vi "AddChannel.vi"(0 "VIRef":refnum<vi>[](array[refnum]), 1 "Name":string="172.16.21.19", 3 "SetCurrent":dbl format="%#.2g", 5 "ADRESS":string[](array[string]), 7 "error in (no error)":errorcluster, 9 "NAME":string[](array[string]), 11 "Address":string="172.16.21.19", 12 "SetVoltage":dbl format="%#.2g") -> (4 "NumRows":i32, 6 "NAMEOut":string[](array[string]), 8 "error out":errorcluster, 10 "ADRESSOut":string[](array[string]), 15 "VIRefOut":refnum<vi>[](array[refnum]))   [LabVIEW 2013]
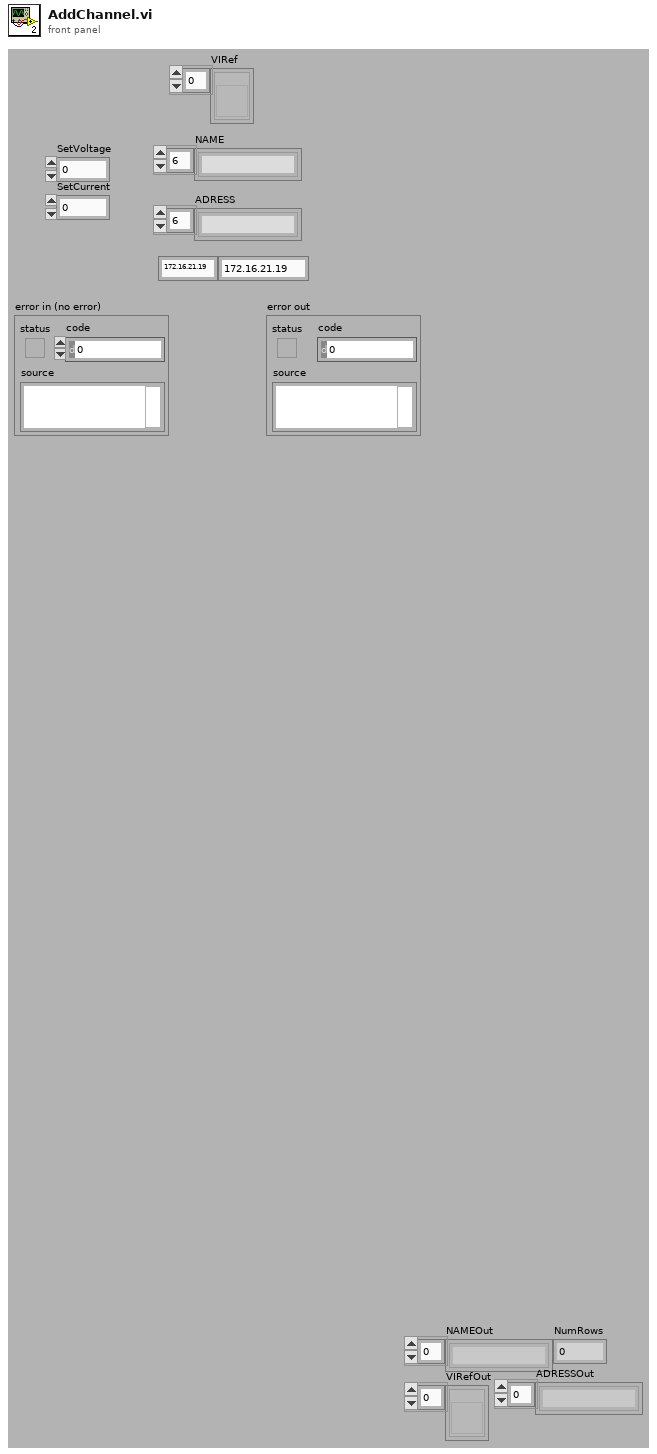
[diagram p1: front panel]
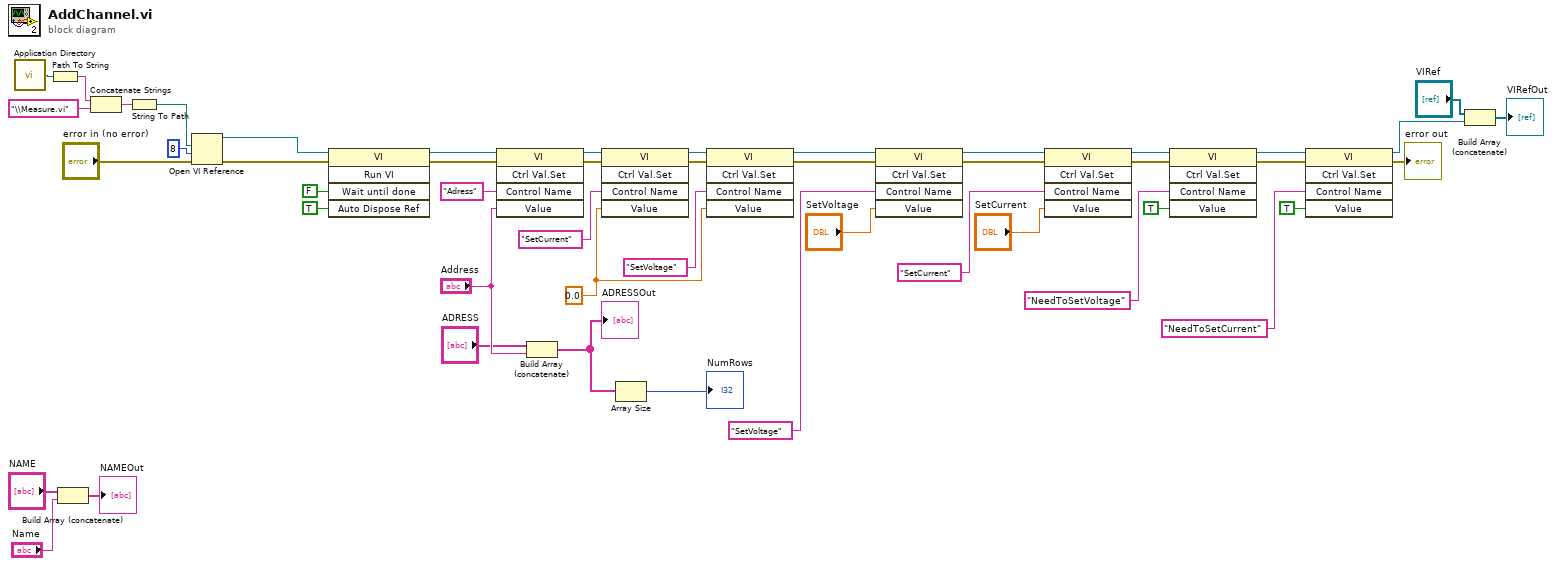
[diagram p0: block diagram]
diagram:
  w28 = 0.0 ("SetCurrent")
  n1 = call <vilib>:"Application Directory.vi"() -> ("Application Directory"=w11:path)
  n2 = Path To String(path=w11) -> (string=w15:string)
  n3 = Build Array (concatenate)("NAME", "Name") -> (→"NAMEOut":string[])
  n4 = Concatenate Strings(w15, "\\Measure.vi" ("string")) -> (w13:string)
  n5 = String To Path(string=w13) -> (path=w12:path)
  n6 = Open VI Reference(vi path=w12, options=8, error in (no error)="error in (no error)") -> (vi reference=w44:refnum<vi>, error out=w47:errorcluster)  [unwired: 1 in, 2 out]
  n7 = invoke class="VI" method="Run VI"(reference=w44, error in=w47, "Wait until done"=FALSE ("Wait Until Done"), "Auto Dispose Ref"=TRUE ("Auto Dispose Reference")) -> (reference out=w41:refnum<vi>, error out=w31:errorcluster)  [unwired: 1 in, 3 out]
  n8 = invoke class="VI" method="Ctrl Val.Set"(reference=w41, error in=w31, "Control Name"="Adress", "Value"="Address") -> (reference out=w33:refnum<vi>, error out=w30:errorcluster)  [unwired: 1 in, 3 out]
  n9 = Build Array (concatenate)("ADRESS", "Address") -> (w39:string[])
  "ADRESSOut" <- w39
  n10 = invoke class="VI" method="Ctrl Val.Set"(reference=w33, error in=w30, "Control Name"="SetCurrent", "Value"=w28) -> (reference out=w32:refnum<vi>, error out=w29:errorcluster)  [unwired: 1 in, 3 out]
  n11 = Array Size(array=w39) -> (size(s)=→"NumRows":i32)
  n12 = invoke class="VI" method="Ctrl Val.Set"(reference=w32, error in=w29, "Control Name"="SetVoltage", "Value"=w28) -> (reference out=w23:refnum<vi>, error out=w22:errorcluster)  [unwired: 1 in, 3 out]
  n13 = invoke class="VI" method="Ctrl Val.Set"(reference=w23, error in=w22, "Control Name"="SetVoltage", "Value"="SetVoltage") -> (reference out=w27:refnum<vi>, error out=w26:errorcluster)  [unwired: 1 in, 3 out]
  n14 = invoke class="VI" method="Ctrl Val.Set"(reference=w27, error in=w26, "Control Name"="SetCurrent", "Value"="SetCurrent") -> (reference out=w8:refnum<vi>, error out=w7:errorcluster)  [unwired: 1 in, 3 out]
  n15 = invoke class="VI" method="Ctrl Val.Set"(reference=w8, error in=w7, "Control Name"="NeedToSetVoltage", "Value"=TRUE ("ConnectChannel")) -> (reference out=w4:refnum<vi>, error out=w3:errorcluster)  [unwired: 1 in, 3 out]
  n16 = invoke class="VI" method="Ctrl Val.Set"(reference=w4, error in=w3, "Control Name"="NeedToSetCurrent", "Value"=TRUE ("ConnectChannel")) -> (reference out=w2:refnum<vi>, error out=→"error out":errorcluster)  [unwired: 1 in, 3 out]
  n17 = Build Array (concatenate)("VIRef", w2) -> (→"VIRefOut":refnum<vi>[])
